vi "Configure Synchronize Source.vi"(8 "error in":errorcluster, 9 "source selection":T1(ring), 10 "channel":T2(ring), 11 "VISA resource name":refnum<visa-resource-name>) -> (0 "error out":errorcluster, 3 "VISA resource out":refnum<visa-resource-name>)   [LabVIEW 2018, in "Suita SPAW7000.lvlib"]
uses:
  <instrlib>/Suita SPAW7000/Suita SPAW7000.lvlib
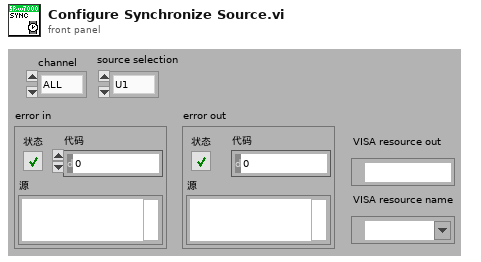
[diagram p1: front panel]
types:
  T1 = enum16{"U1", "U2", "U3", "U4", "U5", "U6", "U7", "I1", "I2", "I3", "I4", "I5", "I6", "I7", "EXT", "NONE"}
  T2 = enum16{"ALL", "ELEM1", "ELEM2", "ELEM3", "ELEM4", "ELEM5", "ELEM6", "ELEM7", "SIGMA", "SIGMB", "SIGMC"}
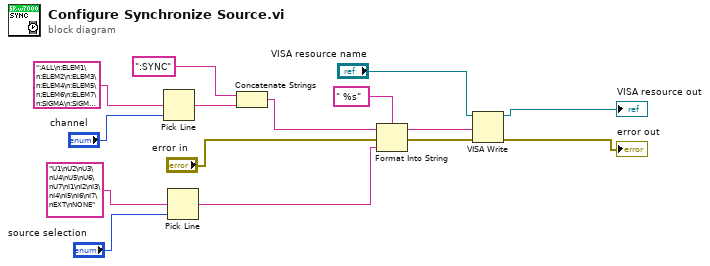
[diagram p0: block diagram]
diagram:
  n1 = Pick Line(multi-line string=":ALL\n:ELEM1\n:ELEM2\n:ELEM3\n:ELEM4\n:ELEM5\n:ELEM6\n:ELEM7\n:SIGMA\n:SIGMB\n:SIGMC", line index="channel") -> (output string=w11:string)  [unwired: 1 in]
  n2 = Pick Line(multi-line string="U1\nU2\nU3\nU4\nU5\nU6\nU7\nI1\nI2\nI3\nI4\nI5\nI6\nI7\nEXT\nNONE", line index="source selection") -> (output string=w8:string)  [unwired: 1 in]
  n3 = Concatenate Strings(":SYNC", w11) -> (w9:string)
  n4 = Format Into String(format string=" %s" ("格式字符串"), initial string=w9, error in="error in", w8) -> (resulting string=w5:string, error out=w6:errorcluster)
  n5 = VISA Write(VISA resource name="VISA resource name", write buffer=w5, error in (no error)=w6) -> (VISA resource name out=→"VISA resource out":refnum<visa-resource-name>, error out=→"error out":errorcluster)  [unwired: 1 out]
